vi "DisableNagle.vi"(8 "error in":errorcluster, 10 "TCP_NODELAY":bool, 11 "connection ID":refnum<k5>) -> (0 "error out":errorcluster, 3 "connID out":refnum<k5>)   [LabVIEW 2014]
doc: "code from https://knowledge.ni.com/KnowledgeArticleDetails?id=kA00Z0000019NZfSAM&l=en-IL"
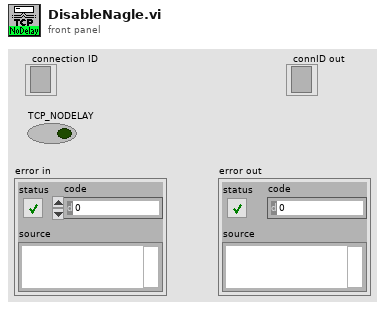
[diagram p1: front panel]
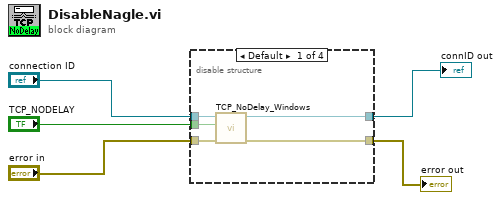
[diagram p0: block diagram]
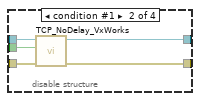
[diagram p2: hidden frame]
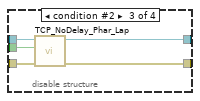
[diagram p3: hidden frame]
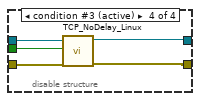
[diagram p4: hidden frame]
diagram:
  n1 = disable-structure shown="Default" {
    disable-tunnel: [w10 w14 w19 w21] -> w1
    disable-tunnel: [w9 w13 w18 w22] -> w2
    disable-tunnel: "connection ID" -> [w8 w12 w17 w24]
    disable-tunnel: "TCP_NODELAY" -> [w7 w11 w16 w23]
    disable-tunnel: "error in" -> [w6 w15 w20 w25]
    frame condition #0 {
      n2 = call "TCP_NoDelay_Windows.vi"("error in (no error)"=w6, "TCP_NODELAY (true)"=w7, "connID"=w8) -> ("error out"=w10:errorcluster, "connID 2"=w9:refnum<k5>)  [unwired: 3 in]
    }
    frame condition #1 {
      n3 = call "TCP_NoDelay_VxWorks.vi"("error in (no error)"=w15, "TCP_NODELAY (true)"=w11, "connID"=w12) -> ("error out"=w14:errorcluster, "connID 2"=w13:refnum<k5>)  [unwired: 3 in]
    }
    frame condition #2 {
      n4 = call "TCP_NoDelay_Phar_Lap.vi"("error in (no error)"=w20, "TCP_NODELAY (true)"=w16, "connID"=w17) -> ("error out"=w19:errorcluster, "connID 2"=w18:refnum<k5>)  [unwired: 3 in]
    }
    frame condition #3 (active) {
      n5 = call "TCP_NoDelay_Linux.vi"("error in (no error)"=w25, "TCP_NODELAY (true)"=w23, "connID"=w24) -> ("error out"=w21:errorcluster, "connID 2"=w22:refnum<k5>)  [unwired: 3 in]
    }
  }
  "connID out" <- w2
  "error out" <- w1
